vi "poly_control_ref_from_name_self_multi.vi"(8 "error in":errorcluster caption="Error in (no error)", 9 "control names":string[](array[string])) -> (0 "error out":errorcluster, 1 "control refs":refnum<vi>[](array[refnum]), 4 "found?":bool[](array[boolean]))   [LabVIEW 2015]
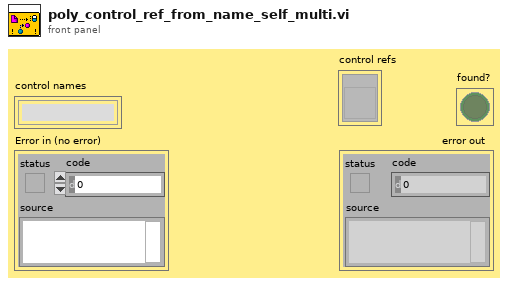
[diagram p1: front panel]
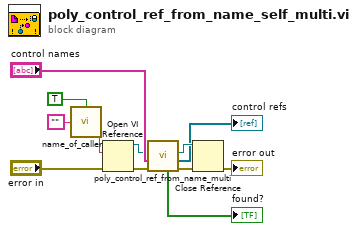
[diagram p0: block diagram]
diagram:
  n1 = call "name_of_caller.vi"("is in inlined vi? (F)"=TRUE, "name of caller in"="") -> ("name of caller out"=w11:string)  [unwired: 2 in]
  n2 = Open VI Reference(vi path=w11, error in (no error)="error in") -> (vi reference=w7:refnum<vi>, error out=w4:errorcluster)  [unwired: 4 in]
  n3 = call "poly_control_ref_from_name_multi.vi"("error in (no error)"=w4, "control names"="control names", "vi ref"=w7) -> ("error out"=w3:errorcluster, "ctrl refs"=→"control refs":refnum<vi>[], "vi ref dup"=w6:refnum<vi>, "found?"=→"found?":bool[])  [unwired: 5 in]
  n4 = Close Reference(reference=w6, error in (no error)=w3) -> (error out=→"error out":errorcluster)
